vi "Unique_D.vi"(11 "1D Array In":dbl[](array[numeric])) -> (3 "Boolean":bool)   [LabVIEW 2009]
uses:
  UniqueLast_D.vi
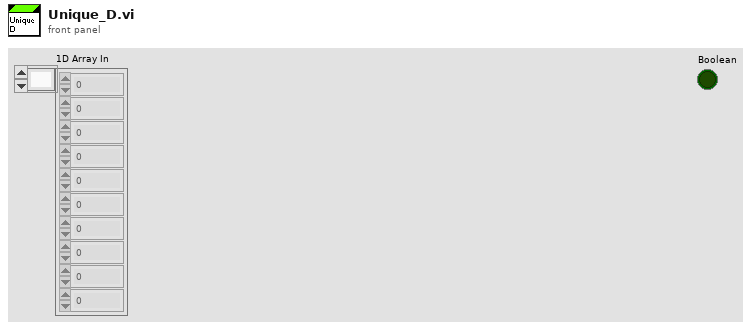
[diagram p1: front panel]
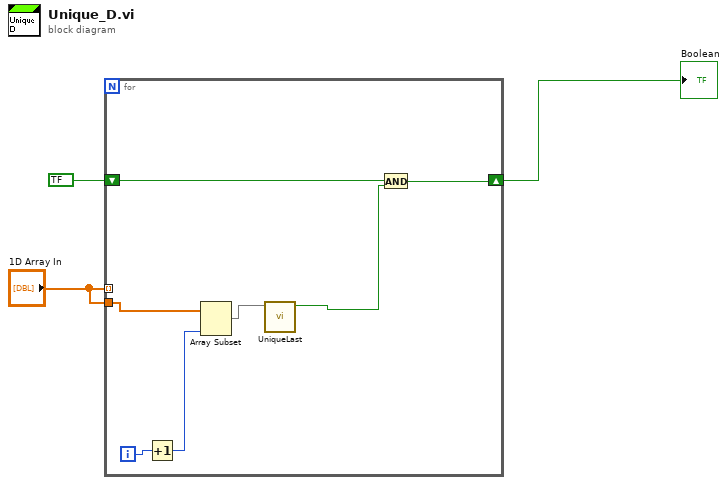
[diagram p0: block diagram]
diagram:
  n1 = for {
    shift-right: [w8] -> w2
    shift-left: bool ? -> [w7]
    tunnel: "1D Array In" -> [_] mode=indexing
    tunnel: "1D Array In" -> [w6]
    i -> [w10]
    n2 = Increment(x=w10) -> (x+1=w9:i32)
    n3 = Array Subset(array=w6, length=w9) -> (w5:dbl[])  [unwired: 1 in]
    n4 = call-poly "UniqueLast.vi"("1D Array In"=w5) -> ("Boolean"=w4:bool)  [unwired: 10 in]
    n5 = And(x=w7, y=w4) -> (x .and. y?=w8:bool)
  }
  "Boolean" <- w2
